vi "Write Environment Options.vi"(8 "error in (no error)":errorcluster, 10 "Environment Options":T1, 11 "WebView2 Control in":refnum<class "WebView2 Control.lvclass">) -> (0 "error out":errorcluster, 3 "WebView2 Control out":refnum<class "WebView2 Control.lvclass">)   [LabVIEW 2020, in "WebView2.lvlib" / "WebView2 Control.lvclass"]
uses:
  WebView2 Control.lvclass
  WebView2 Control.lvclass/WebView2 Control.ctl
  Core Env Options.ctl
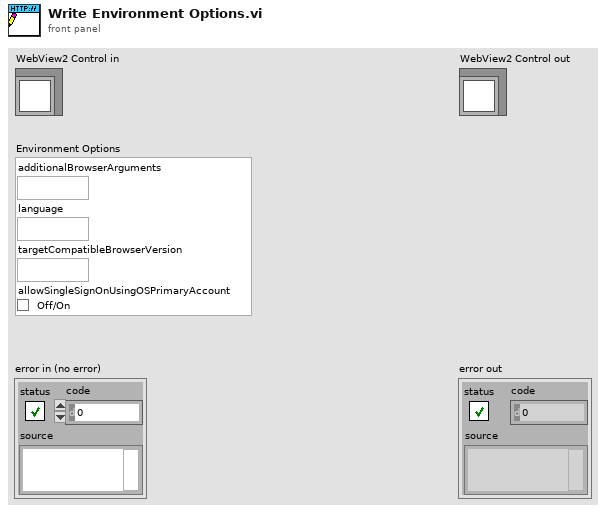
[diagram p1: front panel]
types:
  T1 = typedef "WebView2.lvlib/WebView2 Control.lvclass/Core Env Options.ctl" = cluster{"additionalBrowserArguments":string, "language":string, "targetCompatibleBrowserVersion":string, "allowSingleSignOnUsingOSPrimaryAccount":bool}
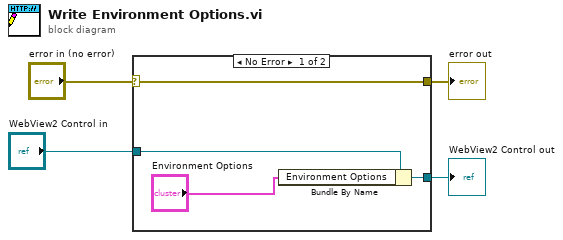
[diagram p0: block diagram]
diagram:
  n1 = case shown="No Error" "error in (no error)" {
    selector: "error in (no error)" -> [w8 w9]
    tunnel: [w8 w9] -> w3
    tunnel: [w6 w10] -> w1
    tunnel: "WebView2 Control in" -> [w7 w10]
    frame No Error {
      n2 = Bundle By Name(cluster=w7, "Environment Options"="Environment Options") -> (w6:refnum<class "WebView2 Control.lvclass">)
    }
    frame Error {
    }
  }
  "error out" <- w3
  "WebView2 Control out" <- w1
